vi "SHIFTER.vi"() -> (8 "SHIFTER DATA":T1={"State"=enum."<Startup>", "User Data"={"Active Item Tag"=""}, "Display Data"={"Current Project Name"="", "Active Icon"=bytes[0]}, "User Parameter Controls"=[], "Framework Data"={"Exit Event"=refnum, "Terminate Error"={"status"=FALSE, "code"=0, "source"=""}}, "Private Data"={"Active Item Tag"="", "Scroll Event"=refnum, "ActiveProject"=refnum, "Active VI"={"App Ref"=refnum, "VI Name"="", "Active Window"=enum."BD", "Icon"=refnum}, "Loaded VI"=refnum, "Collection View Tree"=refnum, "Item View"=refnum, "VI Collection"=refnum}})   [LabVIEW 2013, in "QuickVIew.lvlib"]
uses:
  QuickVIew.lvlib
  TypeDef - SHIFTER.ctl
  VI Collection/VI Collection.lvclass
  <vilib>/LabVIEW Icon API/lv_icon/Classes/Icon/Icon.lvclass
  State Declaration.ctl
  Dependencies.llb/Exit Event Ref.ctl
  Dependencies.llb/TLB`_Dependencies.lvlib
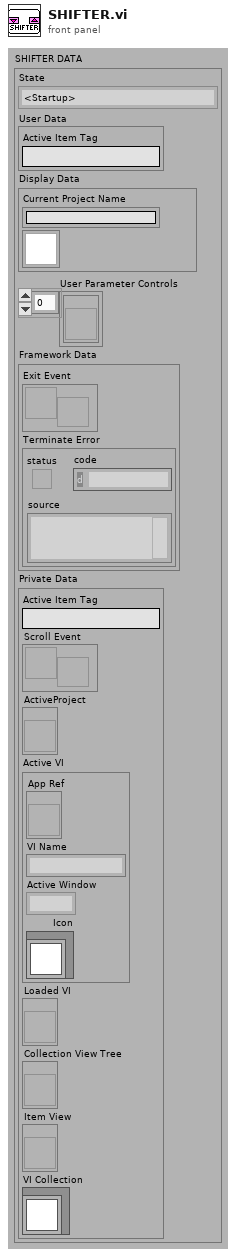
[diagram p1: front panel]
types:
  T1 = typedef "QuickVIew.lvlib/TypeDef - SHIFTER.ctl" = cluster{"State":T2, "User Data":cluster{"Active Item Tag":string}, "Display Data":cluster{"Current Project Name":string, "Active Icon":picture}, "User Parameter Controls":refnum<vi>[], "Framework Data":cluster{"Exit Event":T3, "Terminate Error":errorcluster}, "Private Data":cluster{"Active Item Tag":string, "Scroll Event":refnum<user-event>, "ActiveProject":refnum<vi>, "Active VI":cluster{"App Ref":refnum<vi>, "VI Name":string, "Active Window":enum16{"FP", "BD"}, "Icon":refnum<class "Icon.lvclass">}, "Loaded VI":refnum<vi>, "Collection View Tree":refnum<vi>, "Item View":refnum<vi>, "VI Collection":refnum<class "VI Collection.lvclass">}}
  T2 = typedef "QuickVIew.lvlib/State Declaration.ctl" = enum16{"<Startup>", "Idle", "<Shutdown>", "-", "Viewing"}
  T3 = typedef "QuickVIew.lvlib/TLB`_Dependencies.lvlib/Exit Event Ref.ctl" = refnum<user-event>
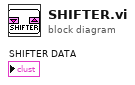
[diagram p0: block diagram]
diagram:
